vi "Frequency Shift.vi"(0 "data in":T1[](array[typedef])=[{"I"=0.0, "Q"=0.0, "overflow"=FALSE}, {"I"=0.0, "Q"=0.0, "overflow"=FALSE}], 9 "input valid":bool, 11 "gen in":refnum<class "niUSRP Tx DSP v2 FPGA.lvclass">, 12 "ready for output (T)":bool=TRUE) -> (4 "data out":T1[](array[typedef]), 10 "output valid":bool, 14 "ready for input":bool, 15 "gen out":refnum<class "niUSRP Tx DSP v2 FPGA.lvclass">)   [LabVIEW 2025, in "niUSRP Tx DSP v2 FPGA.lvclass"]
uses:
  niUSRP Tx DSP v2 FPGA.lvclass
  <instrlib>/_niInstr/DSP/v1/Shared/Public/IQ Data.ctl
  niUSRP Tx DSP v2 FPGA.lvclass/niUSRP Tx DSP v2 FPGA.ctl
  <instrlib>/_niInstr/DSP Control/Interface/v1/FPGA/Frequency Shift/IQ 18-bit/Frequency Shift Interface (IQ 18-bit).lvclass
  <instrlib>/_niInstr/DSP/v1/Shared/niInstr DSP v1 Shared.lvlib
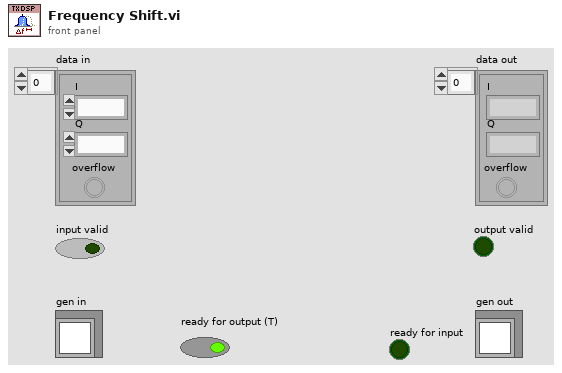
[diagram p1: front panel]
types:
  T1 = typedef "niInstr DSP v1 Shared.lvlib/IQ Data.ctl" = cluster{"I":fxp<+/-,18,1>, "Q":fxp<+/-,18,1>, "overflow":bool}
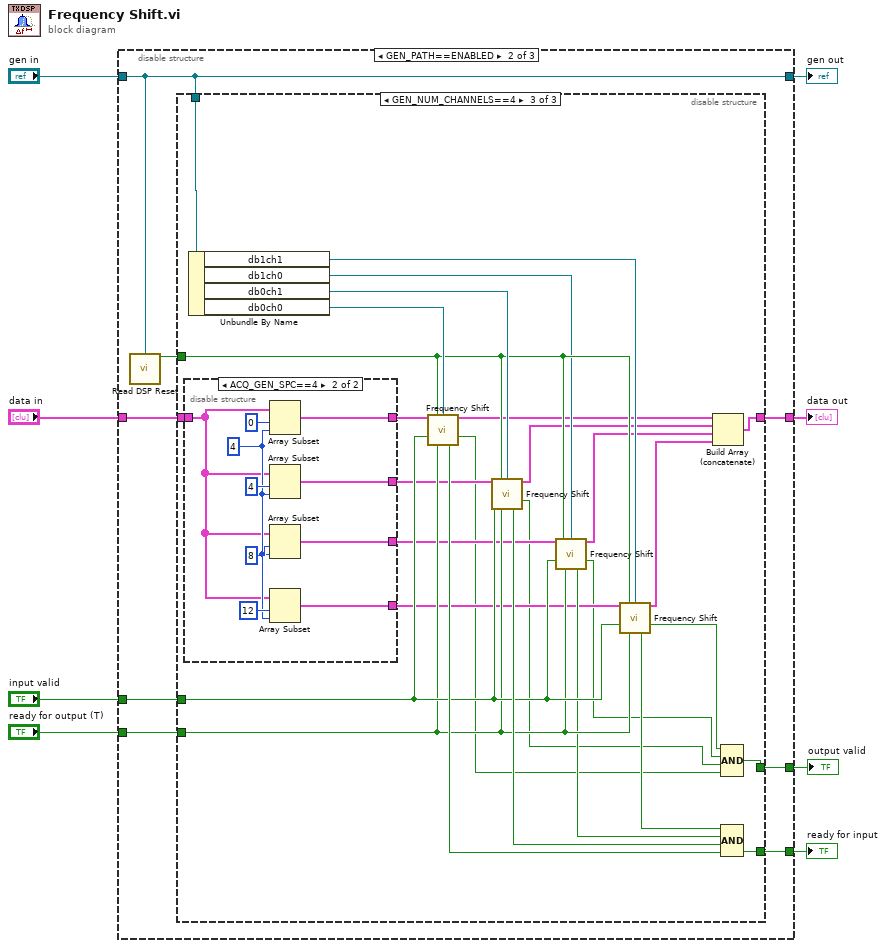
[diagram p0: block diagram]
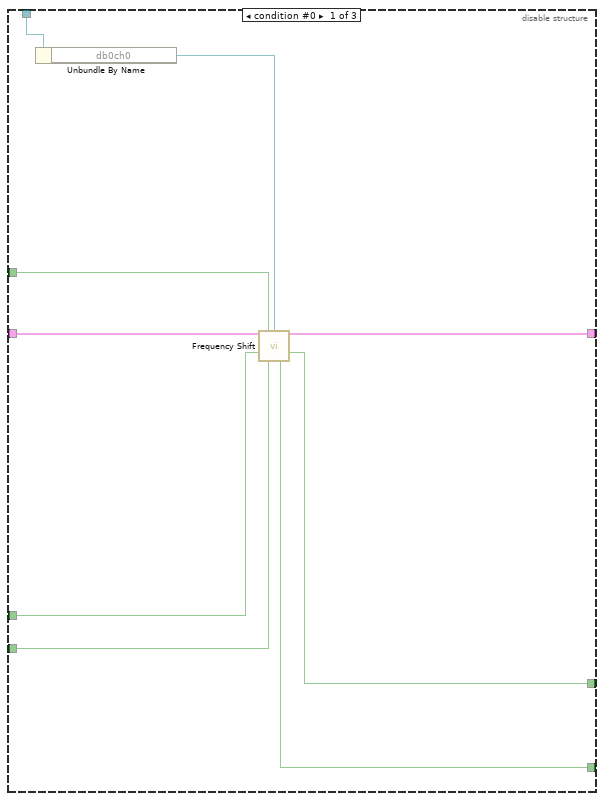
[diagram p3: hidden frame]
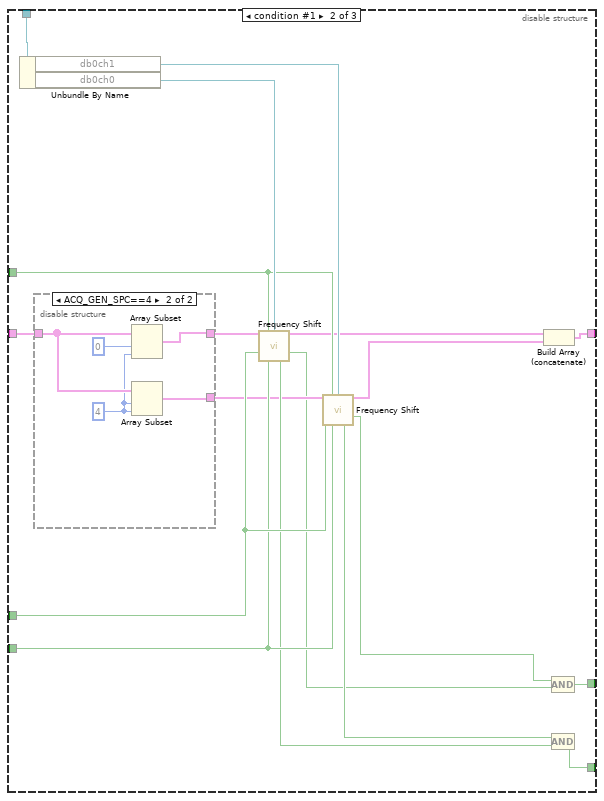
[diagram p4: hidden frame]
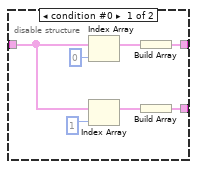
[diagram p5: hidden frame]
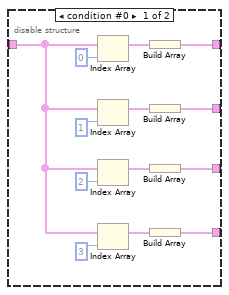
[diagram p6: hidden frame]
diagram:
  n1 = disable-structure shown="GEN_PATH==ENABLED" {
    disable-tunnel: "input valid" -> [_ w16 w107]
    disable-tunnel: "ready for output (T)" -> [_ w15 w108]
    disable-tunnel: [_ w14 w107] -> w6
    disable-tunnel: "gen in" -> [_ w9 w110]
    disable-tunnel: [_ w9 w110] -> w5
    disable-tunnel: "data in" -> [_ w13 w109]
    disable-tunnel: [_ w12 w109] -> w3
    disable-tunnel: [_ w10 w108] -> w2
    frame condition #0 {
      # "IF YOU REACH THIS STATE:\nlabview has failed to propagate the conditional symbol for this structure. to fix this, edit the condition and click OK (typically, no actual changes are necessary)."
    }
    frame condition #1 (active) {
      n2 = call-dynamic "Read DSP Reset.vi"("gen"=w9) -> ("dsp reset"=w11:bool)  [unwired: 14 in]
      n3 = disable-structure shown="GEN_NUM_CHANNELS==4" {
        disable-tunnel: w16 -> [w24 w39 w74]
        disable-tunnel: w15 -> [w23 w38 w72]
        disable-tunnel: [w22 w35 w78] -> w14
        disable-tunnel: w13 -> [w21 w32 w68]
        disable-tunnel: [w20 w34 w77] -> w12
        disable-tunnel: w11 -> [w19 w40 w75]
        disable-tunnel: [w18 w36 w79] -> w10
        disable-tunnel: w9 -> [w17 w42 w82]
        frame condition #0 {
          n4 = Unbundle By Name(w17) -> ("db0ch0"=w25:refnum<class "Frequency Shift Interface (IQ 18-bit).lvclass">)
          n5 = call-dynamic "Frequency Shift.vi"("data in"=w21, "reset"=w19, "frequency shift"=w25, "input valid"=w24, "ready for output (T)"=w23) -> ("data out"=w20:T1[], "output valid"=w22:bool, "ready for input"=w18:bool)  [unwired: 7 in, 1 out]
        }
        frame condition #1 {
          n6 = Unbundle By Name(w42) -> ("db0ch1"=w41:refnum<class "Frequency Shift Interface (IQ 18-bit).lvclass">, "db0ch0"=w43:refnum<class "Frequency Shift Interface (IQ 18-bit).lvclass">)
          n7 = disable-structure shown="ACQ_GEN_SPC==4" {
            disable-tunnel: w32 -> [w46 w53]
            disable-tunnel: [w45 w54] -> w31
            disable-tunnel: [w44 w52] -> w30
            frame condition #0 {
              n8 = Index Array(array=w46, index=0) -> (element=w50:T1)
              n9 = Index Array(array=w46, index=1) -> (element=w48:T1)
              n10 = Build Array(w50) -> (w45:T1[])
              n11 = Build Array(w48) -> (w44:T1[])
            }
            frame condition #1 (active) {
              w51 = 4 ("length")
              n12 = Array Subset(array=w53, index=0, length=w51) -> (w54:T1[])
              n13 = Array Subset(array=w53, index=w51, length=w51) -> (w52:T1[])
            }
          }
          n14 = call-dynamic "Frequency Shift.vi"("data in"=w31, "reset"=w40, "frequency shift"=w43, "input valid"=w39, "ready for output (T)"=w38) -> ("data out"=w29:T1[], "output valid"=w26:bool, "ready for input"=w37:bool)  [unwired: 7 in, 1 out]
          n15 = call-dynamic "Frequency Shift.vi"("data in"=w30, "reset"=w40, "frequency shift"=w41, "input valid"=w39, "ready for output (T)"=w38) -> ("data out"=w28:T1[], "output valid"=w27:bool, "ready for input"=w33:bool)  [unwired: 7 in, 1 out]
          n16 = Build Array (concatenate)(w29, w28) -> (w34:T1[])
          n17 = Compound Arithmetic op=AND(w27, w26) -> (w35:bool)
          n18 = Compound Arithmetic op=AND(w33, w37) -> (w36:bool)
        }
        frame condition #2 (active) {
          n19 = disable-structure shown="ACQ_GEN_SPC==4" {
            disable-tunnel: [w92 w100] -> w67
            disable-tunnel: [w91 w99] -> w66
            disable-tunnel: [w90 w98] -> w65
            disable-tunnel: w68 -> [w85 w101]
            disable-tunnel: [w84 w97] -> w64
            frame condition #0 {
              n20 = Index Array(array=w85, index=0) -> (element=w96:T1)
              n21 = Index Array(array=w85, index=1) -> (element=w94:T1)
              n22 = Index Array(array=w85, index=2) -> (element=w86:T1)
              n23 = Index Array(array=w85, index=3) -> (element=w88:T1)
              n24 = Build Array(w96) -> (w92:T1[])
              n25 = Build Array(w94) -> (w91:T1[])
              n26 = Build Array(w86) -> (w90:T1[])
              n27 = Build Array(w88) -> (w84:T1[])
            }
            frame condition #1 (active) {
              w102 = 4 ("length")
              n28 = Array Subset(array=w101, index=0, length=w102) -> (w100:T1[])
              n29 = Array Subset(array=w101, index=4, length=w102) -> (w99:T1[])
              n30 = Array Subset(array=w101, index=8, length=w102) -> (w98:T1[])
              n31 = Array Subset(array=w101, index=12, length=w102) -> (w97:T1[])
            }
          }
          n32 = Unbundle By Name(w82) -> ("db1ch1"=w69:refnum<class "Frequency Shift Interface (IQ 18-bit).lvclass">, "db1ch0"=w70:refnum<class "Frequency Shift Interface (IQ 18-bit).lvclass">, "db0ch1"=w81:refnum<class "Frequency Shift Interface (IQ 18-bit).lvclass">, "db0ch0"=w83:refnum<class "Frequency Shift Interface (IQ 18-bit).lvclass">)
          n33 = call-dynamic "Frequency Shift.vi"("data in"=w67, "reset"=w75, "frequency shift"=w83, "input valid"=w74, "ready for output (T)"=w72) -> ("data out"=w63:T1[], "output valid"=w56:bool, "ready for input"=w80:bool)  [unwired: 7 in, 1 out]
          n34 = call-dynamic "Frequency Shift.vi"("data in"=w66, "reset"=w75, "frequency shift"=w81, "input valid"=w74, "ready for output (T)"=w72) -> ("data out"=w62:T1[], "output valid"=w57:bool, "ready for input"=w76:bool)  [unwired: 7 in, 1 out]
          n35 = call-dynamic "Frequency Shift.vi"("data in"=w65, "reset"=w75, "frequency shift"=w70, "input valid"=w74, "ready for output (T)"=w72) -> ("data out"=w61:T1[], "output valid"=w58:bool, "ready for input"=w71:bool)  [unwired: 7 in, 1 out]
          n36 = call-dynamic "Frequency Shift.vi"("data in"=w64, "reset"=w75, "frequency shift"=w69, "input valid"=w74, "ready for output (T)"=w72) -> ("data out"=w60:T1[], "output valid"=w59:bool, "ready for input"=w73:bool)  [unwired: 7 in, 1 out]
          n37 = Build Array (concatenate)(w63, w62, w61, w60) -> (w77:T1[])
          n38 = Compound Arithmetic op=AND(w59, w58, w57, w56) -> (w78:bool)
          n39 = Compound Arithmetic op=AND(w73, w71, w76, w80) -> (w79:bool)
        }
      }
    }
    frame condition #2 {
    }
  }
  "data out" <- w3
  "output valid" <- w6
  "ready for input" <- w2
  "gen out" <- w5
